vi "Dispose.vi"(8 "error in (no error)":errorcluster, 11 "ConcreteCreatorA":refnum<class "ConcreteCreatorA.lvclass">) -> (0 "error out":errorcluster)   [LabVIEW 2020, in "FactoryMethod.lvlib" / "ConcreteCreatorA.lvclass"]
uses:
  ConcreteCreatorA.lvclass
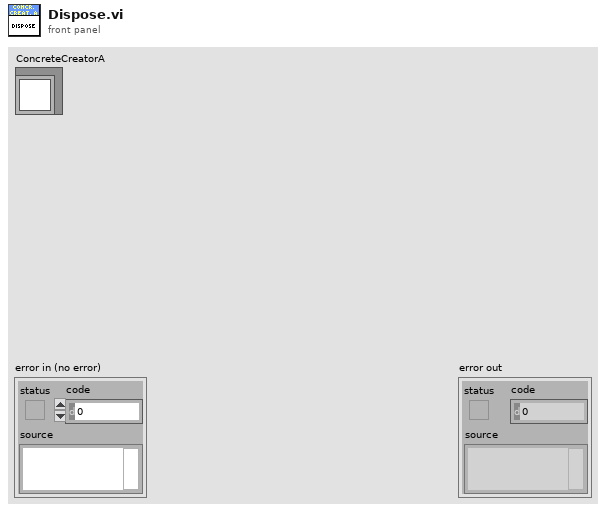
[diagram p1: front panel]
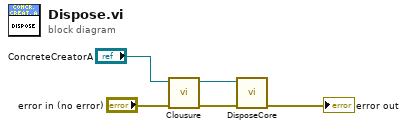
[diagram p0: block diagram]
diagram:
  n1 = call-dynamic "Clousure.vi"("error in (no error)"="error in (no error)", "ConcreteCreatorA in"="ConcreteCreatorA") -> ("error out"=w3:errorcluster, "ConcreteCreatorA out"=w2:refnum<class "ConcreteCreatorA.lvclass">)  [unwired: 8 in]
  n2 = call-dynamic "DisposeCore.vi"("error in (no error)"=w3, "ConcreteCreatorA in"=w2) -> ("error out"=→"error out":errorcluster)  [unwired: 8 in, 1 out]
